vi "c Spark Create.vi"(6 "deviceId":i32, 7 "status":T1, 8 "error in (no error)":errorcluster, 9 "unconfirmedModel":T2 items=["c_Spark_SparkMax"=0, "c_Spark_SparkFlex"=1, "c_Spark_Unknown"=255], 10 "type":T3, 11 "busId":i32) -> (0 "error out":errorcluster, 3 "handle":T4, 5 "status out":T1)   [LabVIEW 2023, in "REVLibDriver.lvlib"]
doc: "c_Spark_handle c_Spark_Create(int deviceId, c_Spark_MotorType type,\n c_Spark_SparkModel unconfirmedModel,\n c_REVLib_ErrorCode* status);"
uses:
  REVLibDriver.lvlib
  lib/libREVLibDriver.so
  Custom Controls/c_Spark_SparkModel.ctl
  Custom Controls/c_Spark_MotorType.ctl
  subvi/RevLibError.ctl
  Custom Controls/c_Spark_handle.ctl
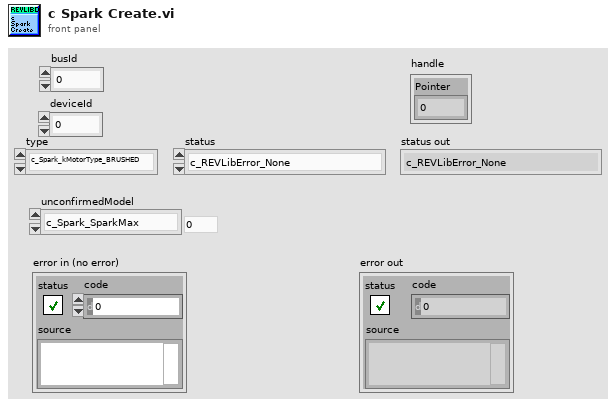
[diagram p1: front panel]
types:
  T1 = typedef "REVLibDriver.lvlib/RevLibError.ctl" = enum16{"c_REVLibError_None", "c_REVLibError_General", "c_REVLibError_CANTimeout", "c_REVLibError_NotImplemented", "c_REVLibError_HAL", "c_REVLibError_CantFindFirmware", "c_REVLibError_FirmwareTooOld", "c_REVLibError_FirmwareTooNew", "c_REVLibError_ParamInvalidID", "c_REVLibError_ParamMismatchType", "c_REVLibError_ParamAccessMode", "c_REVLibError_ParamInvalid", "c_REVLibError_ParamNotImplementedDeprecated", "c_REVLibError_FollowConfigMismatch", "c_REVLibError_Invalid", "c_REVLibError_SetpointOutOfRange", "c_REVLibError_Unknown", "c_REVLibError_CANDisconnected", "c_REVLibError_DuplicateCANId", "c_REVLibError_InvalidCANId", "c_REVLibError_SparkMaxDataPortAlreadyConfiguredDifferently", "c_REVLibError_SparkFlexBrushedWithoutDock", "c_REVLibError_InvalidBrushlessEncoderConfiguration", "c_REVLibError_FeedbackSensorIncompatibleWithDataPortConfig", "c_REVLibError_ParamInvalidChannel", "c_REVLibError_ParamInvalidValue", "c_REVLibError_CannotPersistParametersWhileEnabled", "c_REVLibError_NotReadyToReceiveCommand", "c_REVLibError_NumCodes"}
  T2 = typedef "REVLibDriver.lvlib/c_Spark_SparkModel.ctl" = u16
  T3 = typedef "REVLibDriver.lvlib/c_Spark_MotorType.ctl" = enum16{"c_Spark_kMotorType_BRUSHED", "    c_Spark_kMotorType_BRUSHLESS", "    c_Spark_kNumMotorTypes"}
  T4 = typedef "REVLibDriver.lvlib/c_Spark_handle.ctl" = cluster{"Pointer":u64}
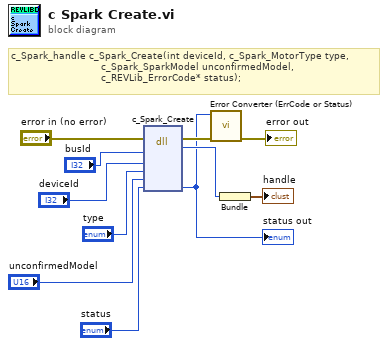
[diagram p0: block diagram]
diagram:
  # "c_Spark_handle c_Spark_Create(int deviceId, c_Spark_MotorType type,\n                              c_Spark_SparkModel unconfirmedModel,\n                              c_REVLib_ErrorCode* status);"
  n1 = dll-call lib="home/systemcore/natinst/lib/libREVLibDriver.so" fn="c_Spark_Create"(error in="error in (no error)", "busID"="busId", "deviceID"="deviceId", "type"="type", "unconfirmedModel"="unconfirmedModel", "status"="status") -> (error out=w6:errorcluster, "return type"=w4:u64, "status"=w1:u32)  [unwired: 6 in, 1 out]
  "status out" <- w1
  n2 = call "Error Converter (ErrCode or Status).vi"("error in (no error)"=w6, "error code"=w1) -> ("error out"=→"error out":errorcluster)  [unwired: 9 in]
  n3 = Bundle("return type"=w4) -> (→"handle":cluster{"return type":u64})  [unwired: 1 in]
